vi "Temporised Pop-up Window.vi"(6 "error window":bool, 8 "error in (no error)":errorcluster, 10 "Timeout":dbl=3.0, 11 "Text":string) -> (0 "error out":errorcluster)   [LabVIEW 2026, in "TALOS.lvlib"]
doc: "Use this VI to create a pop up window that will close if the user press \"OK\" or after the timeout you specify. It is very useful to be sure that an unattended VI will never get blocked because the user is not looking at the screen.\nThe timeout is limited between 1 s and 30 s; the default is 3 s."
uses:
  TALOS.lvlib
  Ancestor/Ancestor/Ancestor.lvclass/Ancestor.ctl
  Generate Error.vi
  FGV/Error Memory/Get Error Description.vi
  Get PC name.vi
  Ancestor/Ancestor/Read ID.vi
  Get Class Name.vi
  <vilib>/Utility/error.llb/Clear Errors.vi
  FGV/Error Memory/Error Memory Core.vi
  <vilib>/AdvancedString/Delimited String to 1D String Array.vi
  <vilib>/AdvancedString/Delimited String to 1D String Array (string).vi
  Circus Root Path.vi
  FGV/Error Memory/Error Crt Lvl checker.vi
  FGV/Error Memory/Error Memory Core.vi/40c8088d-b597-4017-91af-faa98e00292e.vi
  FGV/Error Memory/Error Memory Core.vi/d4a3ab98-063c-4e44-b43d-fbdcfe6c2be2.vi
  Global Memory.vi
  <vilib>/Utility/LVClass/Get LV Class Name.vi
  Is in Packed Library.vi
  Read CSV worksheet.vi
  Global Constants.vi
  <vilib>/Utility/error.llb/General Error Handler.vi
  Error Log.vi
  Ancestor/Ancestor/Ancestor.lvclass
  <vilib>/Comparison/Equal/Equal Functor/Equal Functor.lvclass
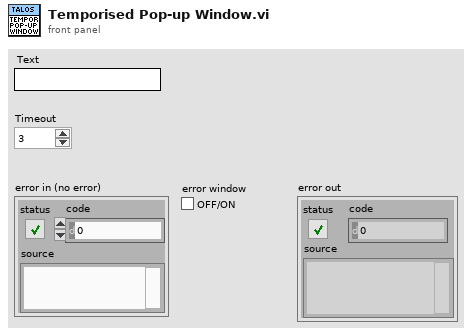
[diagram p1: front panel]
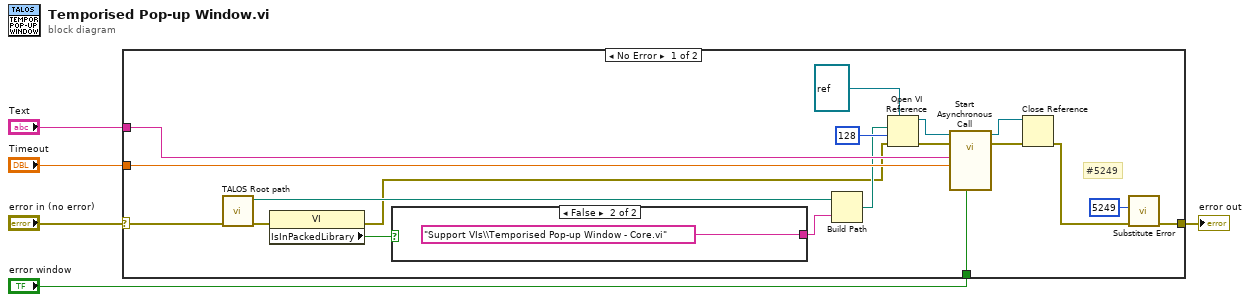
[diagram p0: block diagram]
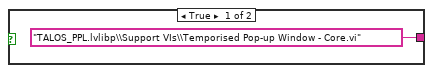
[diagram p2: hidden frame]
diagram:
  n1 = case shown="No Error" "error in (no error)" {
    selector: "error in (no error)" -> [w12 w27]
    tunnel: "Text" -> [w24 _]
    tunnel: "Timeout" -> [w23 _]
    tunnel: [w8 w27] -> w2
    tunnel: "error window" -> [w6 _]
    frame No Error {
      # "#5249"
      n2 = call "TALOS Root path.vi"("error in (no error)"=w12) -> ("error out"=w13:errorcluster, "TALOS Root Path"=w14:path)  [unwired: 9 in]
      n3 = property class="VI"(error in=w13) -> (error out=w10:errorcluster, "IsInPackedLibrary"=w16:bool)  [unwired: 1 in, 1 out]
      n4 = case shown="False" w16 {
        tunnel: ["TALOS_PPL.lvlibp\\Support VIs\\Temporised Pop-up Window - Core.vi" "Support VIs\\Temporised Pop-up Window - Core.vi"] -> w15
        frame True {
        }
        frame False {
        }
      }
      n5 = Build Path(base path=w14, name or relative path=w15) -> (appended path=w11:path)
      n6 = Open VI Reference(type specifier VI Refnum (for type only)=refnum<vi> refnum ("reference"), vi path=w11, options=128, error in (no error)=w10) -> (vi reference=w21:refnum<vi>, error out=w22:errorcluster)  [unwired: 2 in]
      n7 = call-by-ref "Start Asynchronous Call"(reference=w21, error in=w22, "error window"=w6, "Timeout"=w23, "String"=w24) -> (reference out=w18:refnum<vi>, error out=w19:errorcluster)  [unwired: 8 in, 1 out]
      n8 = Close Reference(reference=w18, error in (no error)=w19) -> (error out=w9:errorcluster)
      n9 = call "Substitute Error.vi"("error in (no error)"=w9, "Error Code"=5249) -> ("error out"=w8:errorcluster)  [unwired: 9 in]
    }
    frame Error {
    }
  }
  "error out" <- w2
